vi "DrawGrid.vi"() -> ()   [LabVIEW 2014]
uses:
  TypeDefs/Color.ctl
  TypeDefs/Point3D.ctl
panel:
  in  "Display":T1={"Mode"=enum."Inherit Value", "PointSize"=1.0, "LineWidth"=1.0}
  in  "Color":T2={"Alpha"=1.0, "Color"=16448250} {"Alpha" min=0.0 max=1.0 scale=0.0..1.0}
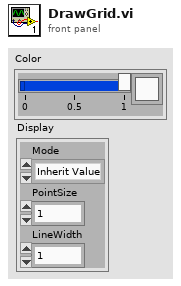
[diagram p1: front panel]
types:
  T1 = cluster{"Mode":enum16{"Inherit Value", "Points", "Wireframe", "Polygons"}, "PointSize":sgl, "LineWidth":sgl}
  T2 = typedef "Color.ctl" = cluster{"Alpha":dbl, "Color":u32}
  T3 = typedef "Point3D.ctl" = cluster{"X":sgl, "Y":sgl, "Z":sgl}
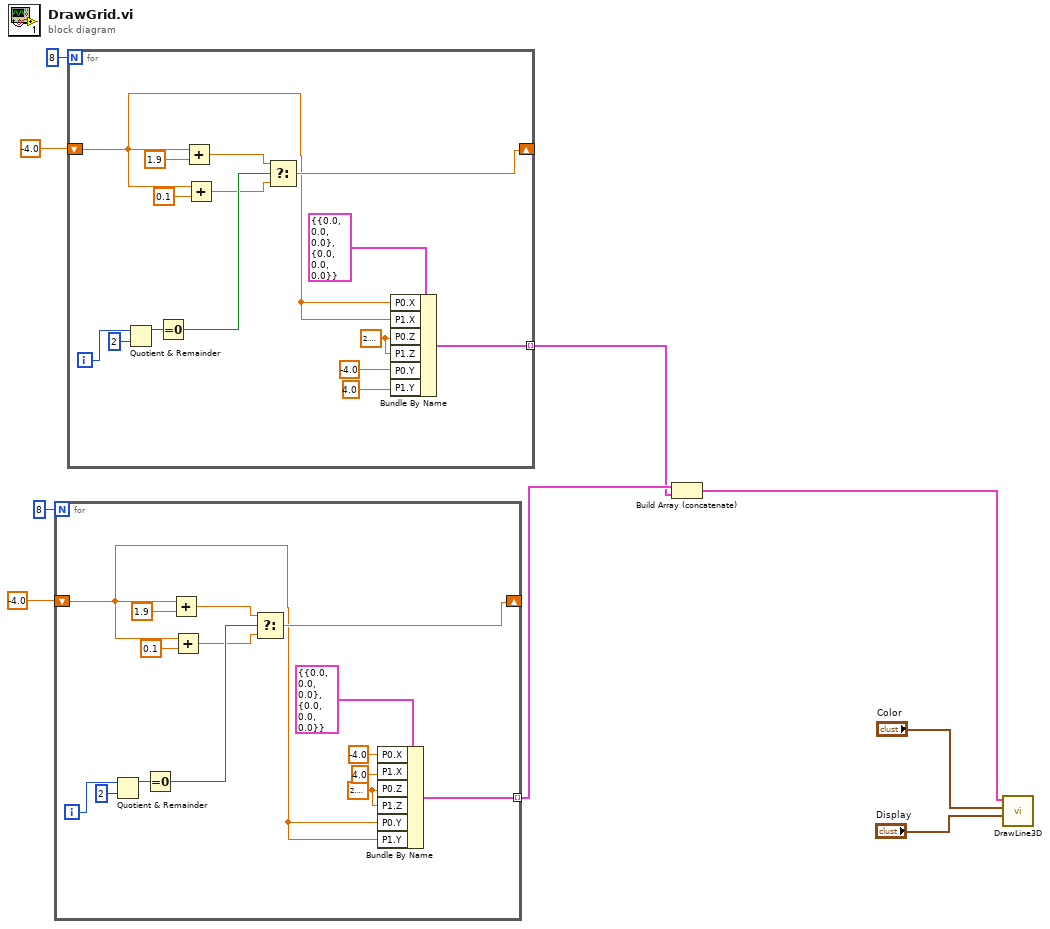
[diagram p0: block diagram]
diagram:
  n1 = for {
    N: 8 -> [_]
    shift-right: [w16] -> _
    shift-left: -4.0 -> [w11]
    tunnel: [w10] -> w3 mode=indexing
    i -> [w24]
    w12 = sgl 2.1 ("P0.Z")
    n2 = Quotient & Remainder(x=w24, y=2) -> (x-y*floor(x/y)=w22:i32)  [unwired: 1 out]
    n3 = Equal To 0?(x=w22) -> (x = 0?=w19:bool)
    n4 = Add(x=w11, y=1.9) -> (x+y=w18:dbl)
    n5 = Add(x=w11, y=0.1) -> (x+y=w17:dbl)
    n6 = Select(t=w18, s=w19, f=w17) -> (s? t:f=w16:dbl)
    n7 = Bundle By Name(cluster=cluster{"P0":T3, "P1":T3} {"P0"={"X"=0.0, "Y"=0.0, "Z"=0.0}, "P1"={"X"=0.0, "Y"=0.0, "Z"=0.0}} ("Line"), "P0.X"=sgl -4.0, "P1.X"=sgl 4.0, "P0.Z"=w12, "P1.Z"=w12, "P0.Y"=w11, "P1.Y"=w11) -> (w10:cluster{"P0":T3, "P1":T3})
  }
  n8 = for {
    N: 8 -> [_]
    shift-right: [w31] -> _
    shift-left: -4.0 -> [w27]
    tunnel: [w28] -> w2 mode=indexing
    i -> [w39]
    w29 = sgl 2.1 ("P0.Z")
    n9 = Quotient & Remainder(x=w39, y=2) -> (x-y*floor(x/y)=w37:i32)  [unwired: 1 out]
    n10 = Equal To 0?(x=w37) -> (x = 0?=w34:bool)
    n11 = Add(x=w27, y=1.9) -> (x+y=w33:dbl)
    n12 = Add(x=w27, y=0.1) -> (x+y=w32:dbl)
    n13 = Select(t=w33, s=w34, f=w32) -> (s? t:f=w31:dbl)
    n14 = Bundle By Name(cluster=cluster{"P0":T3, "P1":T3} {"P0"={"X"=0.0, "Y"=0.0, "Z"=0.0}, "P1"={"X"=0.0, "Y"=0.0, "Z"=0.0}} ("Line"), "P0.X"=w27, "P1.X"=w27, "P0.Z"=w29, "P1.Z"=w29, "P0.Y"=sgl -4.0 ("P0.X"), "P1.Y"=sgl 4.0 ("P1.X")) -> (w28:cluster{"P0":T3, "P1":T3})
  }
  n15 = Build Array (concatenate)(w3, w2) -> (w1:cluster{"P0":T3, "P1":T3}[])
  n16 = call "DrawLine3D.vi"("Display"="Display", "Color"="Color", "Lines"=w1) -> ()  [unwired: 9 in]
